vi "Stimulus Player Loop v2.vi"(8 "Error In":errorcluster, 11 "TopLevel":T1) -> (0 "Error Out":errorcluster)   [LabVIEW 2011]
uses:
  Controls/Top Level Control.ctl
  <vilib>/NI/AMC/Message Queue.ctl
  <vilib>/NI/AMC/Message.ctl
  <vilib>/NI/Tools/Keyed Array/KeyedArray.ctl
  Controls/ListBox Test Record.ctl
  Controls/DVR of CSV Tests Data.ctl
  Controls/CSVs Tests Data.ctl
  Controls/Test Column Data.ctl
  Controls/Options DVR.ctl
  Controls/Options.ctl
  Controls/Stim Player Data.ctl
  <vilib>/NI Veristand/Execution/Workspace/WorkspaceAPI.ctl
  <vilib>/NI Veristand/Execution/SequenceExecutionInterface/Stimulus Profile Session Ref.ctl
  <vilib>/NI Veristand/Execution/ChannelFaultManager/ChannelFaultAPI.ctl
  <vilib>/NI/AMC/Read Termination Message.vi
  <vilib>/NI/AMC/Create Single Message.vi
  <vilib>/NI/AMC/Update Message Routing Info.vi
  Sequence Play/Create Stimulus Session.vi
  Sequence Play/Start Log and Sequence.vi
  GUI Loop/Get Options from DVR.vi
  Sequence Play/Alias or Channel Lookup.vi
  <vilib>/NI/AMC/Globals.vi
  <vilib>/NI/AMC/Send Message.vi
  Sequence Construction/Construct RT Seq Top Level.vi
  <vilib>/NI Veristand/Execution/SequenceExecutionInterface/Get All Sequence Names.vi
  <vilib>/NI Veristand/Execution/SequenceExecutionInterface/Open Stimulus Profile Session.vi
  <vilib>/NI Veristand/Execution/SequenceExecutionInterface/Create Sequence Call.vi
  <vilib>/NI Veristand/Execution/SequenceExecutionInterface/Create Sequence Parameter Assignment.vi
  <vilib>/NI Veristand/Execution/SequenceExecutionInterface/Create Sequence Parameter Assignment (Channel).vi
  <vilib>/NI Veristand/Execution/SequenceExecutionInterface/Register for Stimulus Profile Session Complete Event.vi
  <vilib>/NI Veristand/Execution/SequenceExecutionInterface/Deploy Stimulus Profile Session.vi
  <vilib>/NI Veristand/Execution/Workspace/NI VeriStand - Start Data Logging.vi
  <vilib>/NI Veristand/Execution/Workspace/NI VeriStand - Get System State.vi
  <vilib>/NI Veristand/Execution/Workspace/NI VeriStand - Get Alias List.vi
  <vilib>/NI Veristand/Execution/Workspace/NI VeriStand - Get System Node Channel List.vi
  Sequence Play/Stop Log and Sequence.vi
  <vilib>/NI/AMC/AMC.lvlib
  <vilib>/NI Veristand/Execution/Workspace/NI_VS Workspace ExecutionAPI.lvlib
  <vilib>/NI/Tools/Keyed Array/Tools_KeyedArray.lvlib
  NationalInstruments.VeriStand.ClientAPI
  <vilib>/NI Veristand/Execution/SequenceExecutionInterface/NI_VS Sequence Execution Interface.lvlib
  <vilib>/NI Veristand/Execution/ChannelFaultManager/NI_VS ChannelFault ExecutionAPI.lvlib
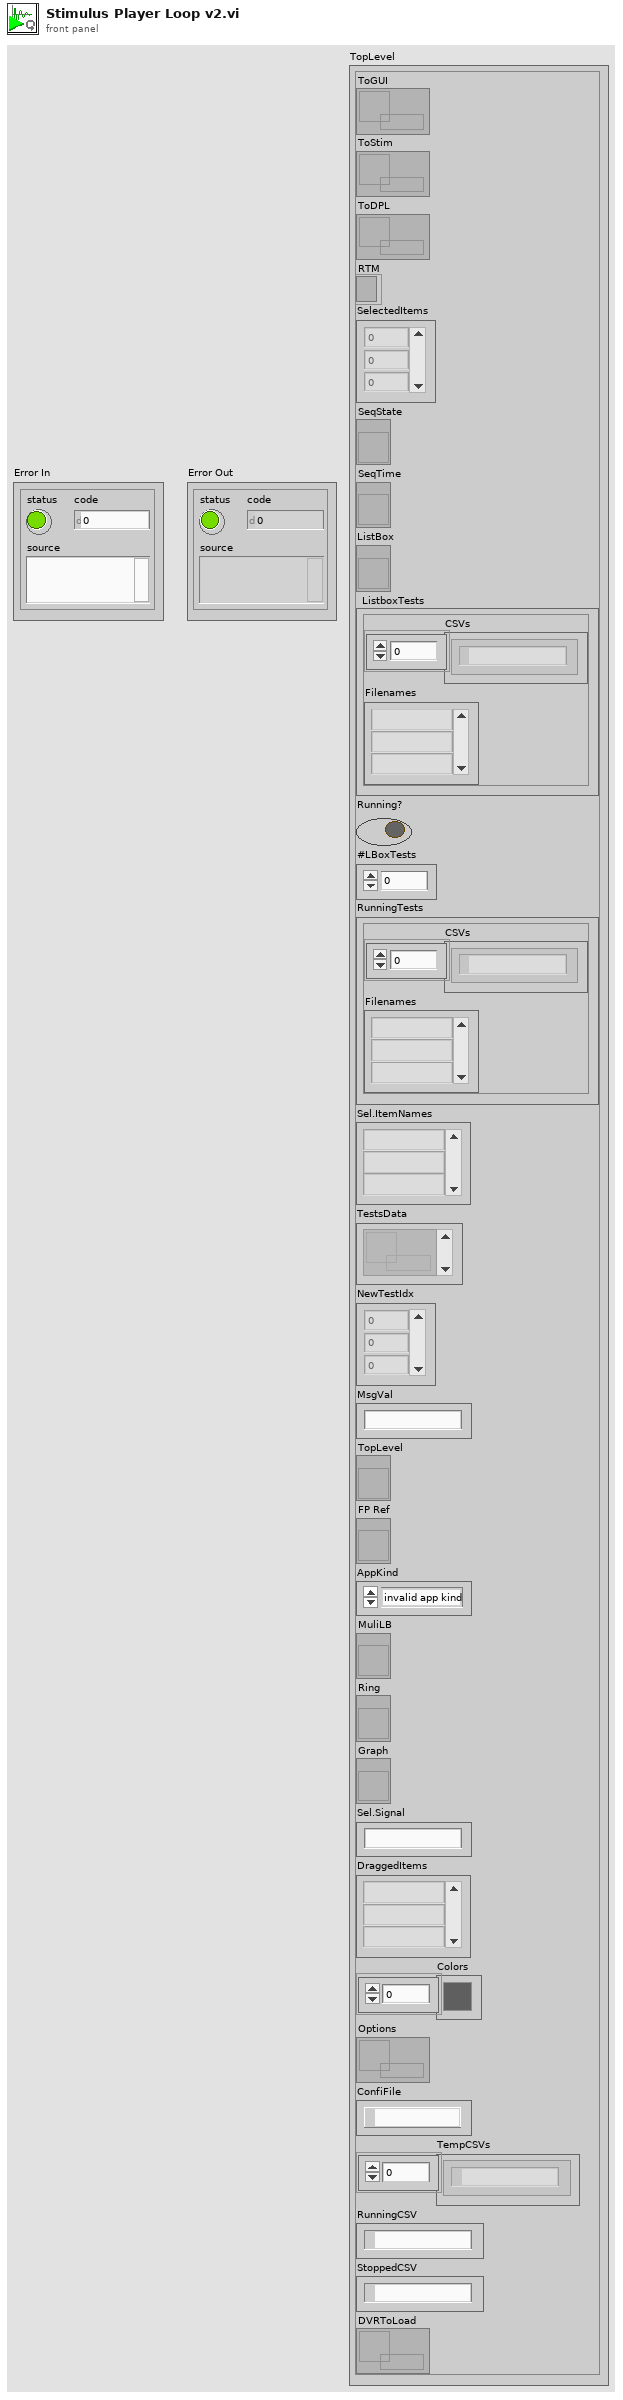
[diagram p1: front panel]
types:
  T1 = typedef "Top Level Control.ctl" = cluster{"ToGUI":T2, "ToStim":T2, "ToDPL":T2, "RTM":refnum<k9>, "SelectedItems":i32[], "SeqState":refnum<vi>, "SeqTime":refnum<vi>, "ListBox":refnum<vi>, "ListboxTests":T3, "Running?":bool, "#LBoxTests":i32, "RunningTests":T3, "Sel.ItemNames":string[], "TestsData":T4[], "NewTestIdx":i32[], "MsgVal":string, "TopLevel":refnum<vi>, "FP Ref":refnum<vi>, "AppKind":enum32{"invalid app kind", "Development System", "Run Time System", "Student Edition", "Embedded LabVIEW", "Evaluation", "Custom"}, "MuliLB":refnum<vi>, "Ring":refnum<vi>, "Graph":refnum<vi>, "Sel.Signal":string, "DraggedItems":string[], "Colors":u32[], "Options":T5, "ConfiFile":path, "TempCSVs":path[], "RunningCSV":path, "StoppedCSV":path, "DVRToLoad":T4}
  T2 = typedef "AMC.lvlib/Message Queue.ctl" = refnum<queue>
  T3 = typedef "ListBox Test Record.ctl" = cluster{"CSVs":path[], "Filenames":string[]}
  T4 = typedef "DVR of CSV Tests Data.ctl" = refnum<data-value>
  T5 = typedef "Options DVR.ctl" = refnum<data-value>
  T6 = typedef "Stim Player Data.ctl" = cluster{"TopLevel":T1, "Wks":T7, "CSV":path, "TestRec":T8, "RTSeq":path, "ParamDefaults":string[][], "SeqCache":path, "StimSess":T10, "SeqName":string, "StimStopped?":bool, "AllStimStopped?":bool, "ChannelFault":T11, "FlatTestRec":string}
  T7 = typedef "NI_VS Workspace ExecutionAPI.lvlib/WorkspaceAPI.ctl" = refnum<k24>
  T8 = typedef "CSVs Tests Data.ctl" = cluster{"Test Data":T9[], "CsvPath":path, "LogPath":path, "Pass?":bool, "Error":errorcluster}
  T9 = typedef "Test Column Data.ctl" = cluster{"Chn":string, "ExpVals":dbl[], "TimeStamps":i64[], "NegTol":dbl, "PosTol":dbl}
  T10 = typedef "NI_VS Sequence Execution Interface.lvlib/Stimulus Profile Session Ref.ctl" = refnum<k24>
  T11 = typedef "NI_VS ChannelFault ExecutionAPI.lvlib/ChannelFaultAPI.ctl" = refnum<k24>
  T12 = typedef "NI_VS Sequence Execution Interface.lvlib/Session Event Ref.ctl" = cluster{"Event Callback":refnum<k27>, "User Event Ref":refnum<user-event>, "Event Registration Refnum":refnum<event-registration>}
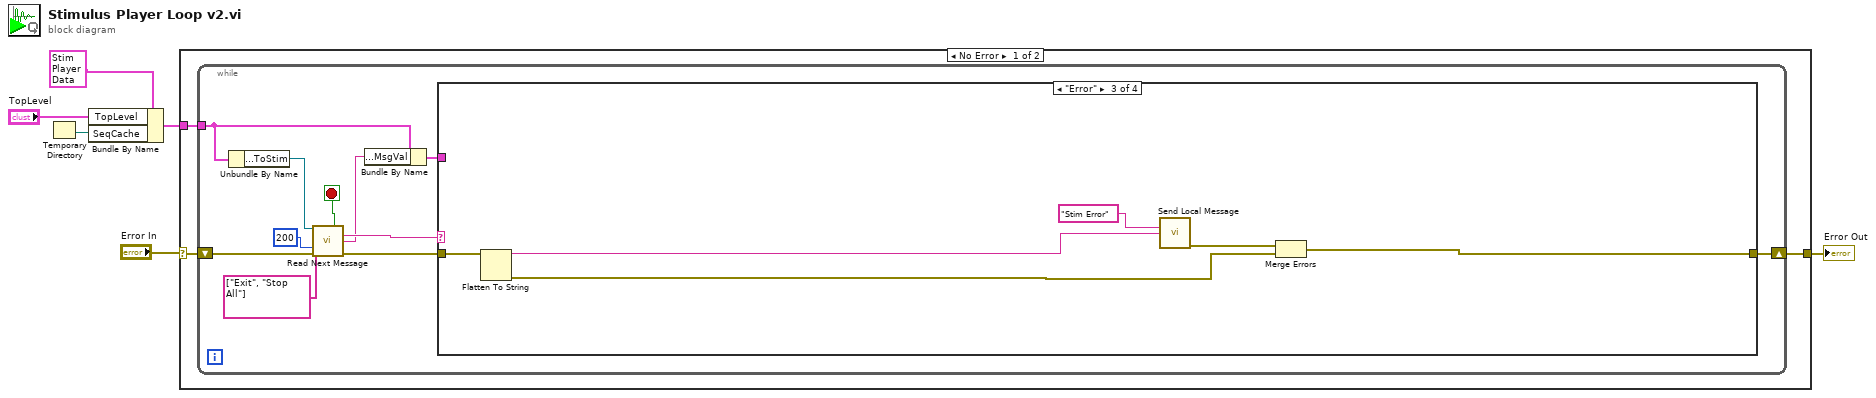
[diagram p0: block diagram]
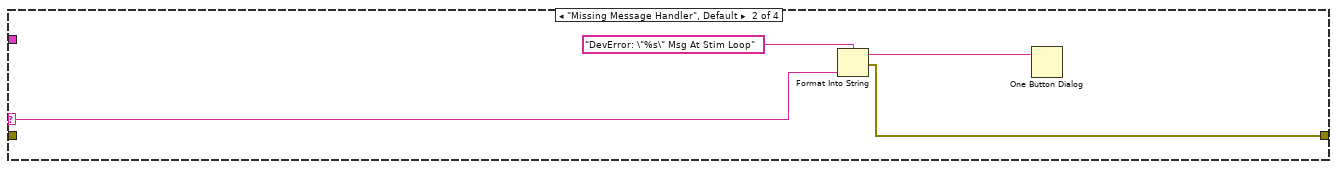
[diagram p3: hidden frame]
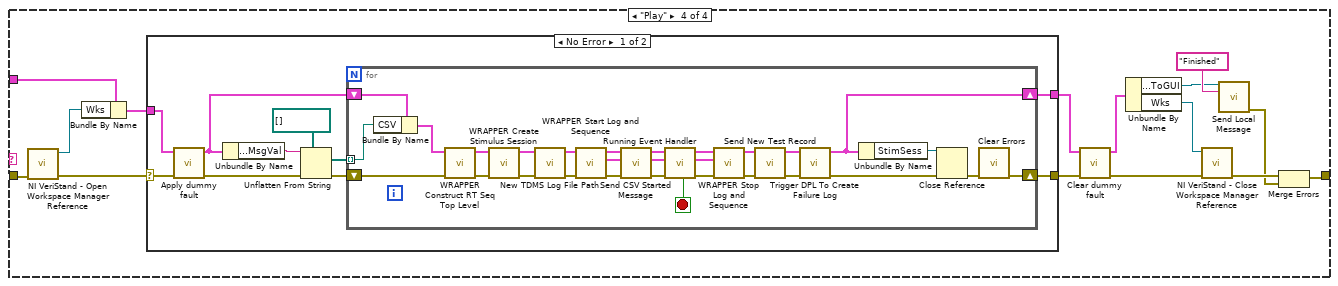
[diagram p4: hidden frame]
diagram:
  n1 = Temporary Directory() -> (w2:path)
  n2 = Bundle By Name(cluster=T6 {"TopLevel"={"ToGUI"=refnum, "ToStim"=refnum, "ToDPL"=refnum, "RTM"=refnum, "SelectedItems"=[], "SeqState"=refnum, "SeqTime"=refnum, "ListBox"=refnum, "ListboxTests"={"CSVs"=[], "Filenames"=[]}, "Running?"=FALSE, "#LBoxTests"=0, "RunningTests"={"CSVs"=[], "Filenames"=[]}, "Sel.ItemNames"=[], "TestsData"=[], "NewTestIdx"=[], "MsgVal"="", "TopLevel"=refnum, "FP Ref"=refnum, "AppKind"=enum."invalid app kind", "MuliLB"=refnum, "Ring"=refnum, "Graph"=refnum, "Sel.Signal"="", "DraggedItems"=[], "Colors"=[], "Options"=refnum, "ConfiFile"=path "", "TempCSVs"=[], "RunningCSV"=path "", "StoppedCSV"=path "", "DVRToLoad"=refnum}, "Wks"=refnum, "CSV"=path "", "TestRec"={"Test Data"=[], "CsvPath"=path "", "LogPath"=path "", "Pass?"=FALSE, "Error"={"status"=FALSE, "code"=0, "source"=""}}, "RTSeq"=path "", "ParamDefaults"=[], "SeqCache"=path "", "StimSess"=refnum, "SeqName"="", "StimStopped?"=FALSE, "AllStimStopped?"=FALSE, "ChannelFault"=refnum, "FlatTestRec"=""} ("Stim Player Data"), "TopLevel"="TopLevel", "SeqCache"=w2) -> (w3:T6)
  n3 = case shown="No Error" "Error In" {
    selector: "Error In" -> [w8 w88]
    tunnel: [w7 w88] -> w5
    tunnel: w3 -> [w9 _]
    frame No Error {
      n4 = while {
        tunnel: w9 -> [w13]
        shift-right: [w14] -> w7
        shift-left: w8 -> [w20]
        stop <- w18 stop-if-true
        n5 = Unbundle By Name(w13) -> ("TopLevel.ToStim"=w15:T2)
        n6 = call <vilib>:"Read Next Message.vi"("message queue in"=w15, "termination list ([Exit])"=string[] ["Exit", "Stop All"] ("Termination List ([Exit])"), "timeout (1 ms)"=200 ("timeout (1ms)"), "error in"=w20) -> ("exit process?"=w18:bool, "message name"=w17:string, "message value"=w12:string, "error out"=w16:errorcluster)  [unwired: 4 in, 4 out]
        n7 = Bundle By Name(cluster=w13, "TopLevel.MsgVal"=w12) -> (w11:T6)
        n8 = case shown="\"Error\"" w17 {
          selector: w17 -> [_ w22 _ _]
          tunnel: w16 -> [w21 _ w29 w42]
          tunnel: [w21 w23 w26 w45] -> w14
          tunnel: w11 -> [_ _ _ w38]
          frame "", "Exit", "Stop All" {
          }
          frame "Missing Message Handler", Default {
            n9 = Format Into String(format string="DevError: \"%s\" Msg At Stim Loop" ("message"), w22) -> (resulting string=w25:string, error out=w23:errorcluster)  [unwired: 2 in]
            n10 = One Button Dialog(message=w25) -> ()  [unwired: 2 out]
          }
          frame "Error" {
            n11 = Flatten To String(anything=w29) -> (data string=w31:string, error out=w27:errorcluster)  [unwired: 3 in, 1 out]
            n12 = call <vilib>:"Send Local Message.vi"("message name"="Stim Error" ("Message Name"), "message value"=w31) -> ("error out"=w28:errorcluster)  [unwired: 11 in, 2 out]
            n13 = Merge Errors(w28, w27) -> (w26:errorcluster)
          }
          frame "Play" {
            n14 = call <vilib>:"NI VeriStand - Open Workspace Manager Reference.vi"("error in (no error)"=w42) -> ("error out"=w39:errorcluster, "WorkspaceManager"=w41:T7)  [unwired: 9 in]
            n15 = Bundle By Name(cluster=w38, "Wks"=w41) -> (w40:T6)
            n16 = case shown="No Error" w39 {
              selector: w39 -> [w50 w87]
              tunnel: [w54 w87] -> w35
              tunnel: [w53 w86] -> w34
              tunnel: w40 -> [w48 w86]
              frame No Error {
                n17 = call "Apply dummy fault.vi"("Error In"=w50, "Stim Player Data in"=w48) -> ("Error Out"=w49:errorcluster, "Stim Player Data out"=w47:T6)  [unwired: 8 in]
                n18 = Unbundle By Name(w47) -> ("TopLevel.MsgVal"=w52:string)
                n19 = Unflatten From String(type=path[] [], binary string=w52, error in (no error)=w49) -> (value=w51:path[], error out=w55:errorcluster)  [unwired: 2 in, 1 out]
                n20 = for {
                  tunnel: w51 -> [w81] mode=indexing
                  shift-right: [w84] -> w54
                  shift-left: w55 -> [w80]
                  shift-right: [w58] -> w53
                  shift-left: w47 -> [w82]
                  stop <- w69 stop-if-true
                  n21 = Bundle By Name(cluster=w82, "CSV"=w81) -> (w79:T6)
                  n22 = call "WRAPPER Construct RT Seq Top Level.vi"("Error In"=w80, "Stim Player Data In"=w79) -> ("Error Out"=w77:errorcluster, "Stim Player Data Out"=w78:T6)  [unwired: 8 in]
                  n23 = call "WRAPPER Create Stimulus Session.vi"("Error In"=w77, "Stim Player Data In"=w78) -> ("Error Out"=w76:errorcluster, "Stim Player Data Out"=w75:T6)  [unwired: 8 in]
                  n24 = call "New TDMS Log File Path.vi"("Error In"=w76, "Stim Player Data In"=w75) -> ("Error Out"=w74:errorcluster, "Stim Player Data Out"=w73:T6)  [unwired: 8 in]
                  n25 = call "WRAPPER Start Log and Sequence.vi"("error in (no error)"=w74, "Stim Player Data In"=w73) -> ("error out"=w72:errorcluster, "SessComplEvent"=w63:T12, "Stim Player Data Out"=w71:T6)  [unwired: 7 in]
                  n26 = call "Send CSV Started Message.vi"("error in (no error)"=w72, "SessComplEvent"=w63, "Stim Player Data in"=w71) -> ("error out"=w85:errorcluster, "SessComplEvent dup"=w62:T12, "Stim Player Data out"=w70:T6)  [unwired: 6 in]
                  n27 = call "Running Event Handler.vi"("error in (no error)"=w85, "SessComplEvent"=w62, "Stim Player Data In"=w70) -> ("error out"=w68:errorcluster, "SessComplEvent dup"=w61:T12, "Stim Player Data Out"=w67:T6, "AllStimStopped?"=w69:bool)  [unwired: 5 in]
                  n28 = call "WRAPPER Stop Log and Sequence.vi"("error in (no error)"=w68, "SessComplEvent"=w61, "Stim Player Data In"=w67) -> ("error out"=w66:errorcluster, "Stim Player Data Out"=w65:T6)  [unwired: 7 in]
                  n29 = call "Send New Test Record.vi"("error in"=w66, "Stim Player Data In"=w65) -> ("error out"=w60:errorcluster, "Stim Player Data Out"=w59:T6)  [unwired: 8 in]
                  n30 = call "Trigger DPL To Create Failure Log.vi"("error in"=w60, "Stim Player Data In"=w59) -> ("error out"=w57:errorcluster, "Stim Player Data Out"=w58:T6)  [unwired: 8 in]
                  n31 = Unbundle By Name(w58) -> ("StimSess"=w64:T10)
                  n32 = Close Reference(reference=w64, error in (no error)=w57) -> (error out=w83:errorcluster)
                  n33 = call <vilib>:"Clear Errors.vi"("error in (no error)"=w83) -> ("error out"=w84:errorcluster)  [unwired: 6 in]
                }
              }
              frame Error {
              }
            }
            n34 = call "Clear dummy fault.vi"("Error In"=w35, "Stim Player Data in"=w34) -> ("Error Out"=w32:errorcluster, "Stim Player Data out"=w33:T6)  [unwired: 8 in]
            n35 = Unbundle By Name(w33) -> ("TopLevel.ToGUI"=w37:T2, "Wks"=w36:T7)
            n36 = call <vilib>:"NI VeriStand - Close Workspace Manager Reference.vi"("error in (no error)"=w32, "WorkspaceManager"=w36) -> ("error out"=w44:errorcluster)  [unwired: 9 in]
            n37 = call <vilib>:"Send Local Message.vi"("message queue in"=w37, "message name"="Finished" ("message")) -> ("error out"=w43:errorcluster)  [unwired: 11 in, 2 out]
            n38 = Merge Errors(w44, w43) -> (w45:errorcluster)
          }
        }
      }
    }
    frame Error {
    }
  }
  "Error Out" <- w5
